vi "save_out_file_storage.vi"() -> ()   [LabVIEW 2021]
uses:
  <vilib>/Analysis/NI_AALPro.lvlib
  <vilib>/Utility/file.llb/Write Delimited Spreadsheet (DBL).vi
panel:
  out "error":i32
  out "intercept":dbl
  out "slope":dbl
  out "Best Linear Fit":dbl[](array[numeric])
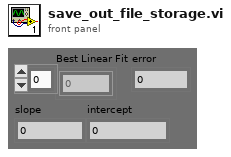
[diagram p1: front panel]
types:
  T1 = enum16{"open", "replace", "create", "open or create", "replace or create", "replace or create with confirmation"}
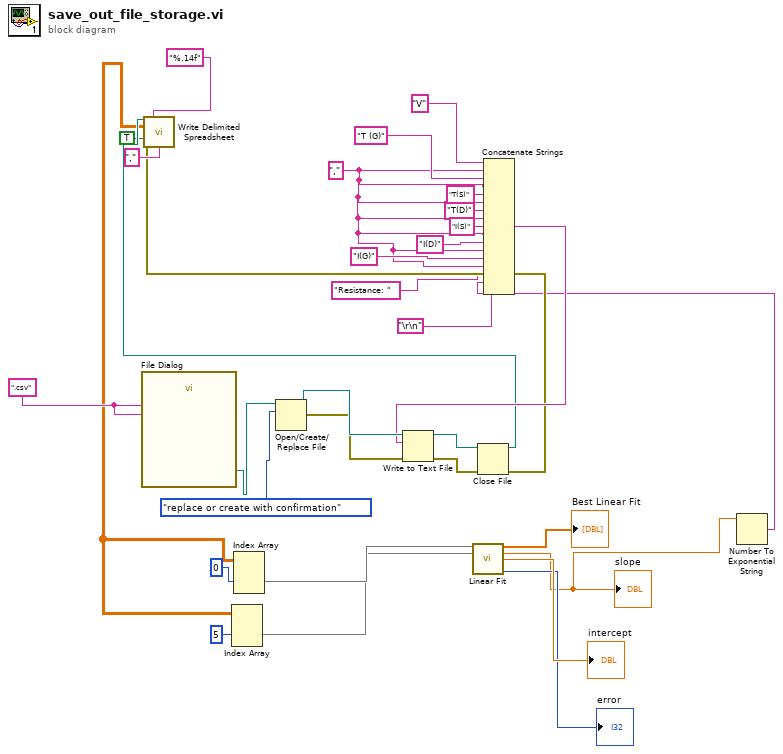
[diagram p0: block diagram]
diagram:
  w6 = "," ("string")
  w25 = ".csv" ("pattern (all files)")
  n1 = call "File Dialog"("pattern (all files)"=w25, "pattern label"=w25) -> ("selected path"=w26:path)  [unwired: 10 in, 3 out]
  n2 = Open/Create/Replace File(file path (use dialog)=w26, operation (0:open)=T1."replace or create with confirmation") -> (refnum out=w31:refnum<file>, error out=w30:errorcluster)  [unwired: 4 in, 1 out]
  n3 = call-poly <vilib>:"Write Delimited Spreadsheet.vi"("file path (dialog if empty)"=w16, "format (%.3f)"="%.14f", "append to file? (new file:F)"=TRUE, "error in (no error)"=w15, "delimiter (\\t)"="," ("delimiter (\\t)")) -> ("2D data"=w1:dbl[][])  [unwired: 8 in, 2 out]
  n4 = Index Array(array=w1, index (dim 1)=5 ("disabled index (col)")) -> (element=w10)  [unwired: 2 in]
  n5 = Index Array(array=w1, index (dim 1)=0 ("disabled index (col)")) -> (element=w12)  [unwired: 2 in]
  n6 = call <vilib>:"Linear Fit.vi"("Y"=w12, "X"=w10) -> ("Best Linear Fit"=→"Best Linear Fit":dbl[], "slope"=w2:dbl, "intercept"=→"intercept":dbl, "error"=→"error":i32)  [unwired: 9 in, 1 out]
  "slope" <- w2
  n7 = Number To Exponential String(number=w2) -> (E-format string=w3:string)  [unwired: 3 in]
  n8 = Concatenate Strings("V" ("string"), w6, "T (G)" ("string"), w6, "T(S)" ("string"), w6, "T(D)" ("string"), w6, "I(S)" ("string"), w6, "I(D)" ("string"), w6, "I(G)" ("string"), w6, "Resistance: " ("string"), w3, "\r\n") -> (w24:string)
  n9 = Write to Text File(file (use dialog)=w31, text=w24, error in=w30) -> (refnum out=w28:refnum<file>, error out=w29:errorcluster)  [unwired: 1 in, 1 out]
  n10 = Close File(refnum=w28, error in=w29) -> (path=w16:path, error out=w15:errorcluster)
